vi "Write File.vi"(8 "error in":errorcluster, 10 "Data In":refnum<class "Data.lvclass">, 11 "File Obs in":refnum<class "PAS File Obs.lvclass">) -> (0 "error out":errorcluster, 3 "File Obs out":refnum<class "PAS File Obs.lvclass">)   [LabVIEW 2014, in "PAS File Obs.lvclass"]
uses:
  PAS File Obs.lvclass
  Main/Controls/pas_data_enum.ctl
  Data/Main/PAS Data.lvclass
  Data/Data.lvclass
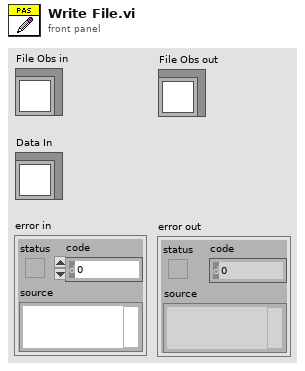
[diagram p1: front panel]
types:
  T1 = typedef "pas_data_enum.ctl" = enum8{"Time", "Ttec", "tecPow", "Spk Position", "Spk Amplification", "Vspan", "Modulation", "Vspk", "Filter", "DC State", "Notes", "O3 Flag", "Raw Flags"}
  T2 = enum16{"big-endian, network order", "native, host order", "little-endian"}
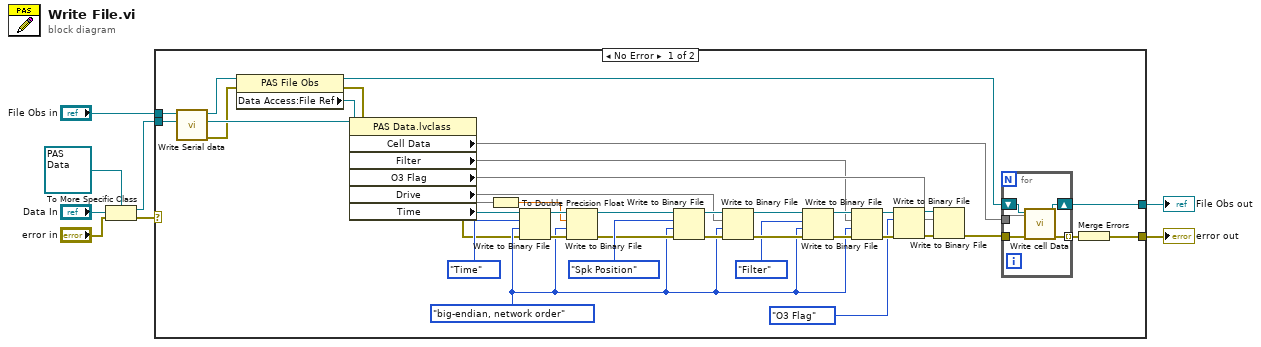
[diagram p0: block diagram]
diagram:
  n1 = To More Specific Class(target class=refnum<class "PAS Data.lvclass"> refnum ("PAS Data"), reference="Data In", error in="error in") -> (specific class reference=w6:refnum<class "PAS Data.lvclass">, error out=w2:errorcluster)
  n2 = case shown="No Error" w2 {
    selector: w2 -> [_ w53]
    tunnel: [w46 w53] -> w1
    tunnel: w6 -> [w26 _]
    tunnel: [w28 w52] -> w5
    tunnel: "File Obs in" -> [w25 w52]
    frame No Error {
      w27 = T2."big-endian, network order" ("byte order (0:big-endian, network order)")
      n3 = call "Write Serial data.vi"("PAS Data In"=w26, "File Obs in"=w25) -> ("error out"=w18:errorcluster, "PAS Data Out"=w24:refnum<class "PAS Data.lvclass">, "File Obs Out"=w21:refnum<class "PAS File Obs.lvclass">)  [unwired: 7 in]
      n4 = property class="PAS File Obs"(reference=w21, error in=w18) -> (reference out=w19:refnum<class "PAS File Obs.lvclass">, error out=w17:errorcluster, "Data Access:File Ref"=w20:refnum<file>)
      n5 = property class="PAS Data.lvclass"(reference=w24, error in=w17) -> (error out=w22:errorcluster, "Cell Data"=w31, "Filter"=w9, "O3 Flag"=w10, "Drive"=w32, "Time"=w30)  [unwired: 1 out]
      n6 = To Double Precision Float(number=w30) -> (double precision float=w29:dbl)
      n7 = Write to Binary File(file (use dialog)=w20, data=pas_data_enum."Time" ("Enum"), error in=w22, 9:w27) -> (refnum out=w43:refnum<file>, error out=w44:errorcluster)  [unwired: 2 in, 1 out]
      n8 = Write to Binary File(file (use dialog)=w43, data=w29, error in=w44, 9:w27) -> (refnum out=w34:refnum<file>, error out=w33:errorcluster)  [unwired: 2 in, 1 out]
      n9 = Write to Binary File(file (use dialog)=w34, data=pas_data_enum."Spk Position" ("Enum"), error in=w33, 9:w27) -> (refnum out=w41:refnum<file>, error out=w42:errorcluster)  [unwired: 2 in, 1 out]
      n10 = Write to Binary File(file (use dialog)=w41, data=w32, error in=w42, 9:w27) -> (refnum out=w38:refnum<file>, error out=w39:errorcluster)  [unwired: 2 in, 1 out]
      n11 = Write to Binary File(file (use dialog)=w38, data=pas_data_enum."Filter" ("Enum"), error in=w39, 9:w27) -> (refnum out=w37:refnum<file>, error out=w36:errorcluster)  [unwired: 2 in, 1 out]
      n12 = Write to Binary File(file (use dialog)=w37, data=w9, error in=w36, 9:w27) -> (refnum out=w14:refnum<file>, error out=w13:errorcluster)  [unwired: 2 in, 1 out]
      n13 = Write to Binary File(file (use dialog)=w14, data=pas_data_enum."O3 Flag" ("Enum"), error in=w13) -> (refnum out=w15:refnum<file>, error out=w16:errorcluster)  [unwired: 3 in, 1 out]
      n14 = Write to Binary File(file (use dialog)=w15, data=w10, error in=w16) -> (error out=w11:errorcluster)  [unwired: 3 in, 2 out]
      n15 = for {
        tunnel: w31 -> [w50]
        tunnel: w11 -> [w51]
        shift-right: [w48] -> w28
        shift-left: w19 -> [w49]
        tunnel: [w47] -> w23 mode=indexing
        n16 = call-dynamic "Write cell Data.vi"("error in"=w51, "PAS Cell Data in"=w50, "PAS File Obs in"=w49) -> ("error out"=w47:errorcluster, "PAS File Obs out"=w48:refnum<class "PAS File Obs.lvclass">)  [unwired: 7 in]
      }
      n17 = Merge Errors(w23) -> (w46:errorcluster)
    }
    frame Error {
    }
  }
  "error out" <- w1
  "File Obs out" <- w5
